vi "Tree to Table Array.vi"(7 "Item Indent":u64, 8 "error in (no error)":errorcluster, 10 "Parent UID":string, 11 "Base Tree in":refnum<class "Base Tree.lvclass">) -> (0 "error out":errorcluster, 2 "Tree Items":T1(array[cluster]), 3 "Base Tree out":refnum<class "Base Tree.lvclass">)   [LabVIEW 2017, in "Browser Core.lvlib" / "Base Tree.lvclass"]
uses:
  Base Tree.lvclass
  Node Classes/Generic Node/Generic Node.lvclass/Generic Node.ctl
  Node Classes/Generic Node/Generic Node.lvclass
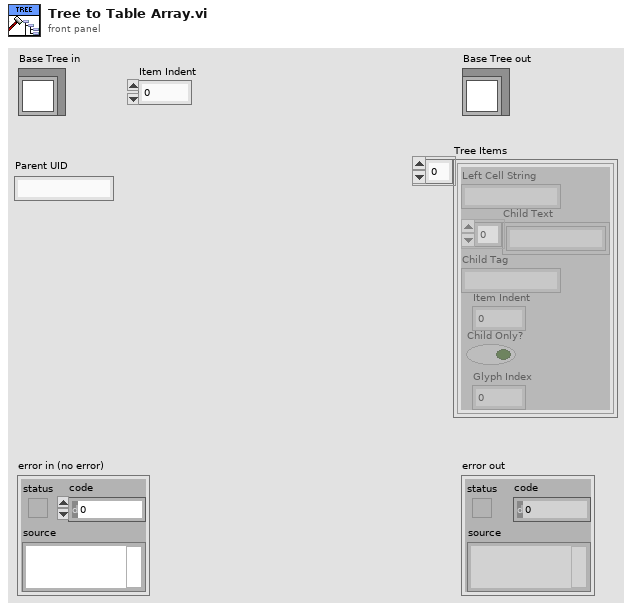
[diagram p1: front panel]
types:
  T1 = cluster{"Left Cell String":string, "Child Text":string[], "Child Tag":string, "Item Indent":i32, "Child Only?":bool, "Glyph Index":i32}[]
  T2 = cluster{"Left Cell String":string, "Child Text":string[], "Child Tag":string, "Item Indent":i32, "Child Only?":bool, "Glyph Index":i32}
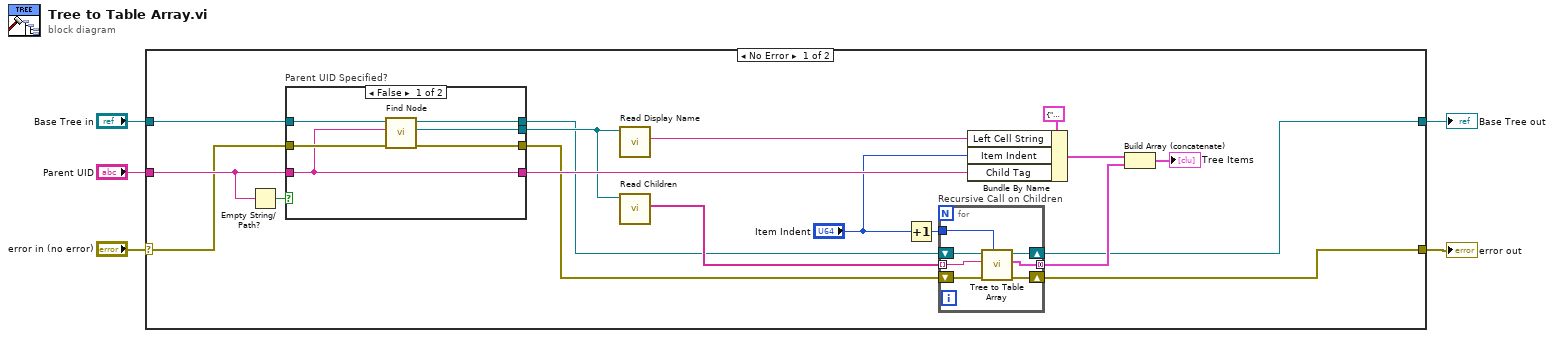
[diagram p0: block diagram]
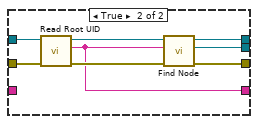
[diagram p2: hidden frame]
diagram:
  n1 = case shown="No Error" "error in (no error)" {
    selector: "error in (no error)" -> [w20 w46]
    tunnel: [w9 w46] -> w4
    tunnel: [w7 w45] -> w2
    tunnel: "Base Tree in" -> [w22 w45]
    tunnel: "Parent UID" -> [w21 _]
    frame No Error {
      n2 = Empty String/Path?(string/path=w21) -> (empty?=w23:bool)
      n3 = case "Parent UID Specified?" shown="False" w23 {
        tunnel: w22 -> [w29 w37]
        tunnel: w21 -> [w24 _]
        tunnel: w20 -> [w28 w34]
        tunnel: [w27 w33] -> w8
        tunnel: [w26 w32] -> w14
        tunnel: [w25 w31] -> w6
        tunnel: [w24 w30] -> w17
        frame False {
          n4 = call-dynamic "Find Node.vi"("error in (no error)"=w28, "UID"=w24, "Base Tree in"=w29) -> ("error out"=w25:errorcluster, "Node"=w26:refnum<class "Generic Node.lvclass">, "Base Tree out"=w27:refnum<class "Base Tree.lvclass">)  [unwired: 5 in, 1 out]
        }
        frame True {
          n5 = call "Read Root UID.vi"("error in (no error)"=w34, "Base Tree in"=w37) -> ("error out"=w35:errorcluster, "Root UID"=w30:string, "Base Tree out"=w36:refnum<class "Base Tree.lvclass">)  [unwired: 7 in]
          n6 = call-dynamic "Find Node.vi"("error in (no error)"=w35, "UID"=w30, "Base Tree in"=w36) -> ("error out"=w31:errorcluster, "Node"=w32:refnum<class "Generic Node.lvclass">, "Base Tree out"=w33:refnum<class "Base Tree.lvclass">)  [unwired: 5 in, 1 out]
        }
      }
      n7 = call "Read Display Name.vi"("Generic Node in"=w14) -> ("Display Name"=w16:string)  [unwired: 8 in, 2 out]
      n8 = call "Read Children.vi"("Generic Node in"=w14) -> ("Children"=w13:string[])  [unwired: 8 in, 2 out]
      n9 = Increment(x="Item Indent") -> (x+1=w12:u64)
      n10 = for "Recursive Call on Children" {
        tunnel: w13 -> [w43] mode=indexing
        tunnel: w12 -> [w42]
        tunnel: [w38] -> w11 mode=concatenating
        shift-right: [w40] -> w9
        shift-left: w6 -> [w41]
        shift-right: [w39] -> w7
        shift-left: w8 -> [w44]
        n11 = call-dynamic "Tree to Table Array.vi"("Item Indent"=w42, "error in (no error)"=w41, "Parent UID"=w43, "Base Tree in"=w44) -> ("error out"=w40:errorcluster, "Tree Items"=w38:T1, "Base Tree out"=w39:refnum<class "Base Tree.lvclass">)  [unwired: 5 in]
      }
      n12 = Bundle By Name(cluster=T2 {"Left Cell String"="", "Child Text"=[], "Child Tag"="", "Item Indent"=0, "Child Only?"=FALSE, "Glyph Index"=0} ("Item"), "Left Cell String"=w16, "Item Indent"="Item Indent", "Child Tag"=w17) -> (w10:T2)
      n13 = Build Array (concatenate)(w10, w11) -> (→"Tree Items":T1)
    }
    frame Error {
    }
  }
  "error out" <- w4
  "Base Tree out" <- w2
